vi "Lock Data.vi"(6 "Wait for Confirmation Timeout [ms] (0=No Wait)":i32, 8 "error in (no error)":errorcluster, 9 "Datum Type":variant, 10 "Datum Name":string, 11 "IModel in":refnum<class "IModel.lvclass">) -> (0 "error out":errorcluster, 3 "IModel out":refnum<class "IModel.lvclass">)   [LabVIEW 2020, in "MVA Framework.lvlib" / "IModel.lvlib" / "IModel.lvclass"]
doc: "锁定数据"
uses:
  IModel.lvclass
  IObserver/IObserver/IObserver.lvclass/IObserver.ctl
  IModel.lvclass/IModel.ctl
  composed-transport/Source/Concrete/NotifierTransport/NotifierTransport.lvclass/NotifierTransport.ctl
  IMediator/IMediator Messages/Lock Publication Msg/Lock Publication Msg.lvclass/Lock Publication Msg.ctl
  composed-af-messages/Source/RoundTripMessage/RoundTripMessage.lvclass/RoundTripMessage.ctl
  <vilib>/ActorFramework/Message Enqueuer/Message Enqueuer.lvclass/Message Enqueuer.ctl
  composed-af-messages/Source/RoundTripMessage/Return Round-Trip Message.vi
  <vilib>/ActorFramework/Message Enqueuer/Enqueue.vi
  composed-transport/Source/Concrete/NotifierTransport/NotifierTransport.lvclass
  IMediator/IMediator Messages/Lock Publication Msg/Lock Publication Msg.lvclass
  composed-af-messages/Source/RoundTripMessage/RoundTripMessage.lvclass
  C:/Program Files/National Instruments/LabVIEW 2020/vi.lib/ActorFramework/Message/Message.lvclass
  <vilib>/ActorFramework/Message Priority Queue/Priority Enqueue.vi
  <vilib>/Utility/error.llb/Error Cluster From Error Code.vi
  IMediator/IPublicationPolicy/IPublicationPolicy.lvclass
  IObserver/IObserver/IObserver.lvclass
  C:/Program Files/National Instruments/LabVIEW 2020/vi.lib/ActorFramework/Actor/Actor.lvclass
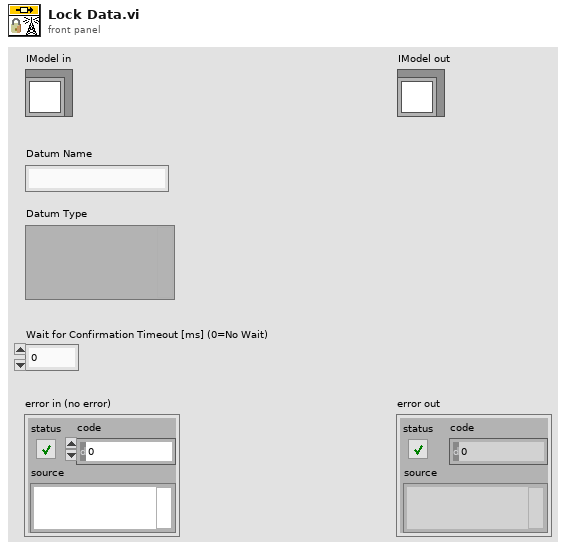
[diagram p1: front panel]
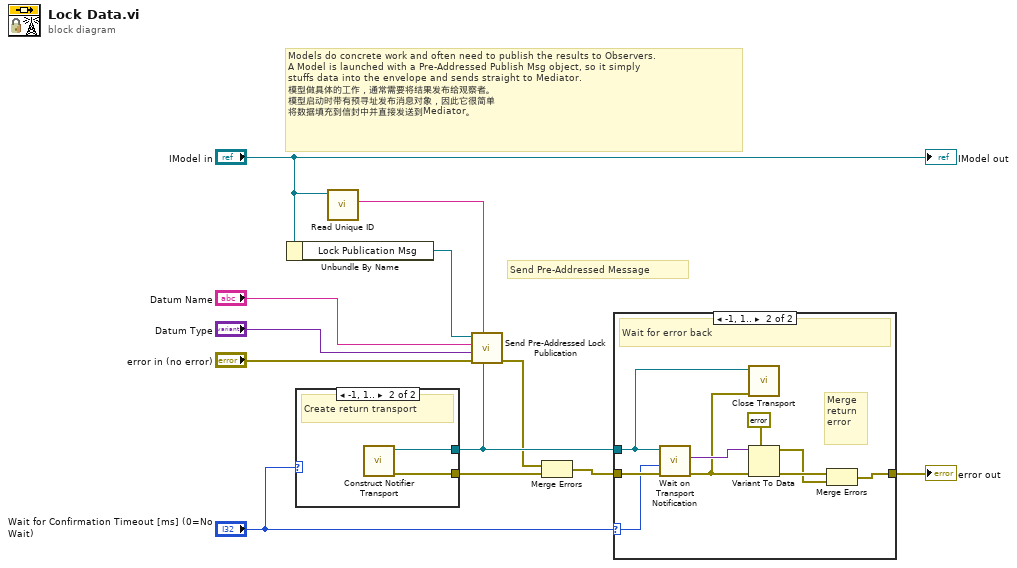
[diagram p0: block diagram]
diagram:
  # "Models do concrete work and often need to publish the results to Observers.\nA Model is launched with a Pre-Addressed Publish Msg object, so it simply\nstuffs data into the envelope and sends straight to Mediator.\n模型做具体的工作，通常需要将结果发布给观察者。\n模型启动时带有预寻址发布消息对象，因此它很简单\n将数据填充到信封中并直接发送到Mediator。"
  # "Send Pre-Addressed Message"
  n1 = Unbundle By Name("IModel in") -> ("Lock Publication Msg"=w12:refnum<class "Lock Publication Msg.lvclass">)
  n2 = case shown="-1, 1.." "Wait for Confirmation Timeout [ms] (0=No Wait)" {
    tunnel: [_ w14] -> w7
    tunnel: [_ w13] -> w4
    frame 0, Default {
      # "Do not handle return error"
    }
    frame -1, 1.. {
      # "Create return transport"
      n3 = call "Construct Notifier Transport.vi"() -> ("error out"=w13:errorcluster, "NotifierTransport"=w14:refnum<class "NotifierTransport.lvclass">)  [unwired: 10 in]
    }
  }
  n4 = call "Read Unique ID.vi"("IObserver In"="IModel in") -> ("Unique ID"=w1:string)  [unwired: 10 in]
  n5 = call "Send Pre-Addressed Lock Publication.vi"("Return Error Transport"=w7, "Publisher ID"=w1, "error in (no error)"="error in (no error)", "Datum Type"="Datum Type", "Datum Name"="Datum Name", "Lock Publication Msg"=w12) -> ("error out"=w2:errorcluster)  [unwired: 5 in]
  n6 = Merge Errors(w2, w4) -> (w3:errorcluster)
  n7 = case shown="-1, 1.." "Wait for Confirmation Timeout [ms] (0=No Wait)" {
    selector: "Wait for Confirmation Timeout [ms] (0=No Wait)" -> [_ w23]
    tunnel: w7 -> [_ w16]
    tunnel: [w15 w19] -> w6
    tunnel: w3 -> [w15 w24]
    frame 0, Default {
      # "No wait"
    }
    frame -1, 1.. {
      # "Merge\nreturn\nerror"
      # "Wait for error back"
      n8 = call "Wait on Transport Notification.vi"("error in (no error)"=w24, "Timeout In ms (-1)"=w23, "NotifierTransport"=w16) -> ("error out"=w17:errorcluster, "Data"=w22:variant)  [unwired: 6 in, 1 out]
      n9 = call-dynamic "Close Transport.vi"("error in (no error)"=w17, "NotifierTransport"=w16) -> ()  [unwired: 9 in, 1 out]
      n10 = Variant To Data(error in=w17, type=errorcluster {"status"=FALSE, "code"=0, "source"=""} ("error constant"), Variant=w22) -> (data=w18:errorcluster, error out=w21:errorcluster)
      n11 = Merge Errors(w21, w18) -> (w19:errorcluster)
    }
  }
  "error out" <- w6
  "IModel out" <- "IModel in"
